vi "Unregister Event.vi"(8 "Error In":errorcluster, 9 "Registrant Address":refnum<class "Message Enqueuer.lvclass">, 10 "Event":refnum<class "Event.lvclass">, 11 "Event Source In":refnum<class "Event Source.lvclass">) -> (0 "Error Out":errorcluster, 3 "Event Source Out":refnum<class "Event Source.lvclass">)   [LabVIEW 2019, in "Event Source.lvlib" / "Event Source.lvclass"]
doc: "This method unregisters a specific Actors Enqueuer from specific Event he is listening to, in this Event Source Actor."
uses:
  Event Source.lvclass
  Event/Event.lvclass
  <resource>/AFDebug/AF Debug.lvlib
  <vilib>/Utility/miscctls.llb/LVMapReplaceAction.ctl
  <vilib>/ActorFramework/Message Enqueuer/Message Enqueuer.lvclass
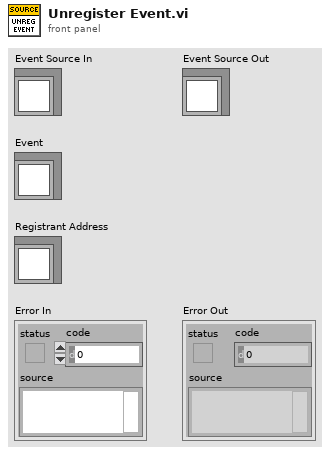
[diagram p1: front panel]
types:
  T1 = typedef "LVMapReplaceAction.ctl" = enum32{"Modify Entry only if found", "Add or Modify Entry", "Delete Entry"}
  T2 = map{string, map{refnum<class "Message Enqueuer.lvclass">, refnum<class "Event Generated Msg.lvclass">}}
  T3 = map{refnum<class "Message Enqueuer.lvclass">, refnum<class "Event Generated Msg.lvclass">}
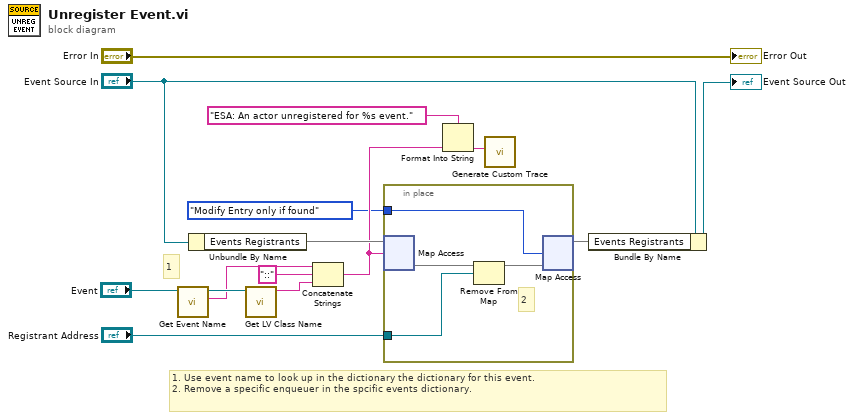
[diagram p0: block diagram]
diagram:
  # "1"
  # "1. Use event name to look up in the dictionary the dictionary for this event.\n2. Remove a specific enqueuer in the spcific events dictionary."
  n1 = call "Get Event Name.vi"("Event In"="Event") -> ("Name"=w10:string, "Event Out"=w13:refnum<class "Event.lvclass">)  [unwired: 9 in]
  n2 = Unbundle By Name("Event Source In") -> ("Events Registrants"=w9:T2)
  n3 = call <vilib>:"Get LV Class Name.vi"("object"=w13) -> ("class name"=w11:string)  [unwired: 9 in, 1 out]
  n4 = Concatenate Strings(w10, "::" ("string"), w11) -> (w8:string)
  n5 = in-place {
    in-place-border: "Registrant Address" -> [w16]
    in-place-border: LVMapReplaceAction."Modify Entry only if found" ("action") -> [w19]
    # "2"
    n6 = in-place-map #1(w9, w8) -> (w18:T3)  [unwired: 1 in, 1 out]
    n7 = Remove From Map(10:w16, 11:w18) -> (3:w17:T3)  [unwired: 2 out]
    n8 = in-place-map #1(w17, w19) -> (w6:T2)  [unwired: 2 out]
  }
  n9 = Format Into String(format string="ESA: An actor unregistered for %s event." ("Custom Action"), w8) -> (resulting string=w14:string)  [unwired: 2 in, 1 out]
  n10 = call <resource>:"Generate Custom Trace.vi"("Custom Action"=w14) -> ()  [unwired: 11 in]
  n11 = Bundle By Name(cluster="Event Source In", "Events Registrants"=w6) -> (→"Event Source Out":refnum<class "Event Source.lvclass">)
  "Error Out" <- "Error In"
